vi "display.vi"(8 "error in (no error)":errorcluster, 11 "CoolDisplay in":refnum<class "CoolDisplay.lvclass">) -> (0 "error out":errorcluster, 3 "CoolDisplay out":refnum<class "CoolDisplay.lvclass">)   [LabVIEW 2018, in "CoolDisplay.lvclass"]
uses:
  CoolDisplay.lvclass
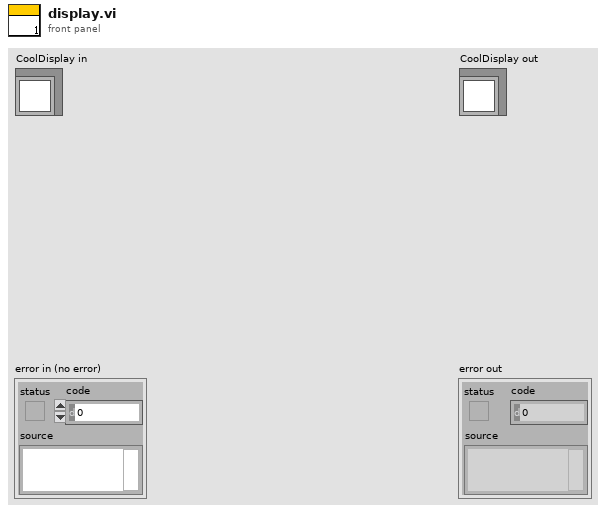
[diagram p1: front panel]
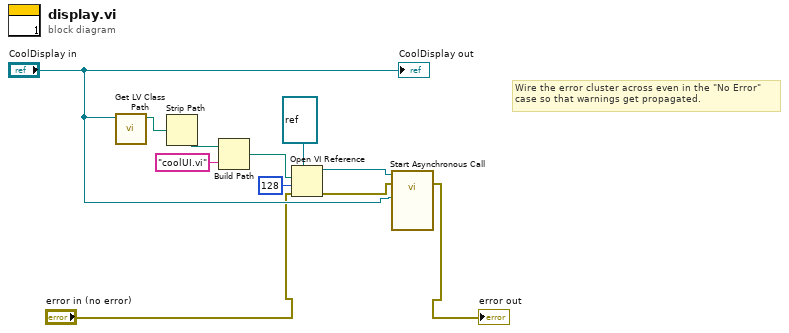
[diagram p0: block diagram]
diagram:
  # "Wire the error cluster across even in the \"No Error\"\ncase so that warnings get propagated."
  n1 = call <vilib>:"Get LV Class Path.vi"("object"="CoolDisplay in") -> ("class path"=w11:path)  [unwired: 9 in, 1 out]
  n2 = Strip Path(path=w11) -> (stripped path=w4:path)  [unwired: 1 out]
  n3 = Build Path(base path=w4, name or relative path="coolUI.vi") -> (appended path=w9:path)
  n4 = Open VI Reference(type specifier VI Refnum (for type only)=refnum<vi> refnum, vi path=w9, options=128, error in (no error)="error in (no error)") -> (vi reference=w7:refnum<vi>, error out=w6:errorcluster)  [unwired: 2 in]
  n5 = call-by-ref "Start Asynchronous Call"(reference=w7, error in=w6, "CoolDisplay.lvclass"="CoolDisplay in") -> (error out=→"error out":errorcluster)  [unwired: 11 in, 1 out]
  "CoolDisplay out" <- "CoolDisplay in"
